vi "Enqueue Unbundled Element.vi"(6 "Priority":T1, 8 "error in":errorcluster, 10 "State":string, 11 "QDMH in":refnum<class "QDMH.lvclass">) -> (0 "error out":errorcluster, 3 "QDMH out":refnum<class "QDMH.lvclass">)   [LabVIEW 2023, in "QDMH.lvlib" / "QDMH.lvclass"]
uses:
  QDMH.lvclass
  Custom Controls/Priority.ctl
  QDMH.lvclass/QDMH.ctl
  Custom Controls/QDMH Message.ctl
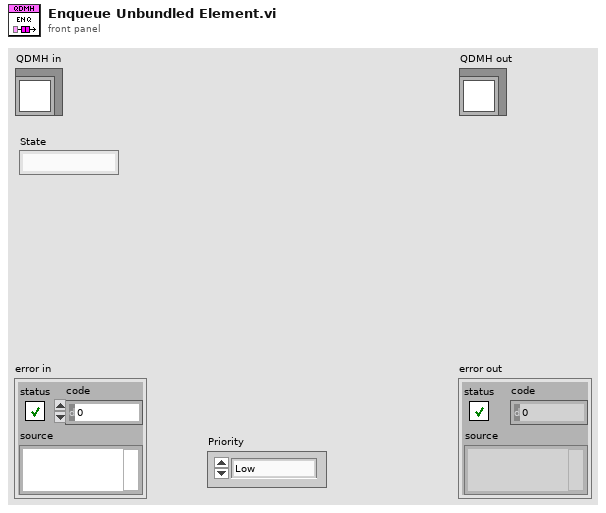
[diagram p1: front panel]
types:
  T1 = typedef "QDMH.lvlib/QDMH.lvclass/Priority.ctl" = enum16{"Low ", "High"}
  T2 = typedef "QDMH.lvlib/QDMH.lvclass/QDMH Message.ctl" = cluster{"State":string, "Data":variant}
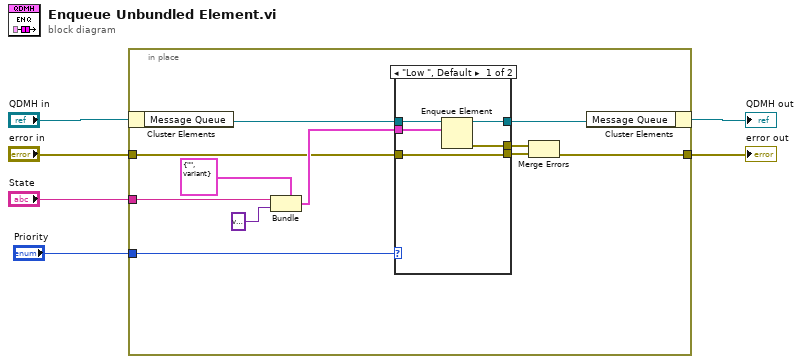
[diagram p0: block diagram]
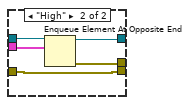
[diagram p2: hidden frame]
diagram:
  n1 = in-place {
    in-place-border: [w8] -> w5
    in-place-border: "error in" -> [w13]
    in-place-border: "State" -> [w12]
    in-place-border: "Priority" -> [w10]
    n2 = in-place-cluster #1("QDMH in") -> ("Message Queue"=w16:refnum<queue>)
    n3 = Bundle(cluster=T2 {"State"="", "Data"=variant} ("Message"), "State"=w12, "Data"=variant) -> (w14:T2)
    n4 = case shown="\"Low \", Default" w10 {
      tunnel: [w22 w26] -> w17
      tunnel: w16 -> [w21 w27]
      tunnel: [w20 w25] -> w15
      tunnel: w14 -> [w19 w24]
      tunnel: w13 -> [w18 w23]
      tunnel: [w18 w23] -> w7
      frame "Low ", Default {
        n5 = Enqueue Element(queue=w21, element=w19) -> (queue out=w22:refnum<queue>, error out=w20:errorcluster)  [unwired: 2 in, 1 out]
      }
      frame "High" {
        n6 = Enqueue Element At Opposite End(queue=w27, element=w24) -> (queue out=w26:refnum<queue>, error out=w25:errorcluster)  [unwired: 2 in, 1 out]
      }
    }
    n7 = Merge Errors(w15, w7) -> (w8:errorcluster)
    n8 = in-place-cluster #1("Message Queue"=w17) -> (→"QDMH out":refnum<class "QDMH.lvclass">)
  }
  "error out" <- w5
